vi "Constants.vi"() -> ()   [LabVIEW 2021, in "DAQ Analog InOut Shared.lvlib"]
doc: "Use this Global VI to access the GUIDs assigned to the page resources of the Custom Device."
uses:
  DAQ Analog InOut Shared.lvlib
panel:
  in  "Tab Control":enum32{"GUIDs", "Constants", "Properties"}(tab)
  in  "Disable DAQ Analog InOut":string="722e37f8-9191-45db-b2f5-cba64aa61de6"
  in  "GUID-AO Section":string="b22111a8-f5d2-4f47-8713-b96c2f7314a2"
  in  "GUID-AI Section":string="c3d51edd-15a0-47f6-a048-5f26947f2f16"
  in  "DAQ Analog InOut":string="6e5ea417-3f02-462b-8a6a-02cbb2ff9692"
  in  "Prop.Output Section":string="Prop.Output Section"
  in  "Prop.Input Section":string="Prop.Input Section"
  in  "Prop.Main":string="Compiled.Settings"
  in  "Compiled.Settings":string="Compiled.Settings"
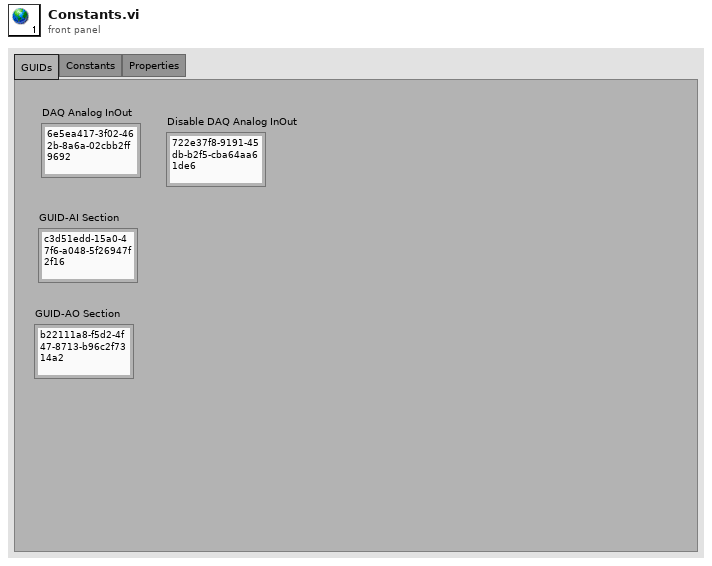
[diagram p1: front panel]
diagram:
